vi "Scan Codes Mapping.vi"() -> ()   [LabVIEW 2021, in "Seq Edit Quick Drop.lvlib"]
uses:
  Seq Edit Quick Drop.lvlib
  Key Code.ctl
panel:
  in  "Scan Codes Mapping":T1[](array[typedef])=[{"Key"="0", "Scan Code"=11}, {"Key"="1", "Scan Code"=2}, {"Key"="2", "Scan Code"=3}, {"Key"="3", "Scan Code"=4}, {"Key"="4", "Scan Code"=5}, {"Key"="5", "Scan Code"=6}, {"Key"="6", "Scan Code"=7}, {"Key"="7", "Scan Code"=8}, {"Key"="8", "Scan Code"=9}, {"Key"="9", "Scan Code"=10}, {"Key"="A", "Scan Code"=30}, {"Key"="B", "Scan Code"=48}, {"Key"="C", "Scan Code"=46}, {"Key"="D", "Scan Code"=32}, {"Key"="E", "Scan Code"=18}, {"Key"="F", "Scan Code"=33}, {"Key"="G", "Scan Code"=34}, {"Key"="H", "Scan Code"=35}, {"Key"="I", "Scan Code"=23}, {"Key"="J", "Scan Code"=36}, {"Key"="K", "Scan Code"=37}, {"Key"="L", "Scan Code"=38}, {"Key"="M", "Scan Code"=50}, {"Key"="N", "Scan Code"=49}, {"Key"="O", "Scan Code"=24}, {"Key"="P", "Scan Code"=25}, {"Key"="Q", "Scan Code"=16}, {"Key"="R", "Scan Code"=19}, {"Key"="S", "Scan Code"=31}, {"Key"="T", "Scan Code"=20}, {"Key"="U", "Scan Code"=22}, {"Key"="V", "Scan Code"=47}, {"Key"="W", "Scan Code"=17}, {"Key"="X", "Scan Code"=45}, {"Key"="Y", "Scan Code"=21}, {"Key"="Z", "Scan Code"=44}]
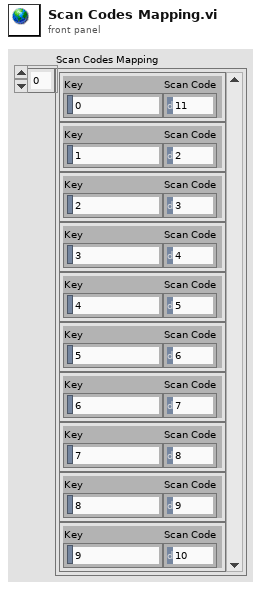
[diagram p1: front panel]
types:
  T1 = typedef "Seq Edit Quick Drop.lvlib/Key Code.ctl" = cluster{"Key":string, "Scan Code":i16}
diagram:
